vi "accelerometerChecker.vi"() -> ()   [LabVIEW 2021]
uses:
  <vilib>/DAQmx/read.llb/DAQmx Read (Analog 1D Wfm NChan NSamp).vi
  <vilib>/DAQmx/create/channels.llb/DAQmx Create Channel (AI-Voltage-Basic).vi
  <vilib>/DAQmx/create/channels.llb/DAQmx Create Channel (AI-Acceleration-Accelerometer).vi
  <vilib>/DAQmx/configure/timing.llb/DAQmx Timing (Sample Clock).vi
  <vilib>/DAQmx/miscellaneous.llb/DAQmx Fill In Error Info.vi
  <resource>/objmgr/daqmx.rc
panel:
  out "data 4":dynamicdata(graph) caption="data"
  out "data 3":dynamicdata(graph) caption="data"
  out "data 2":dynamicdata(graph) caption="data"
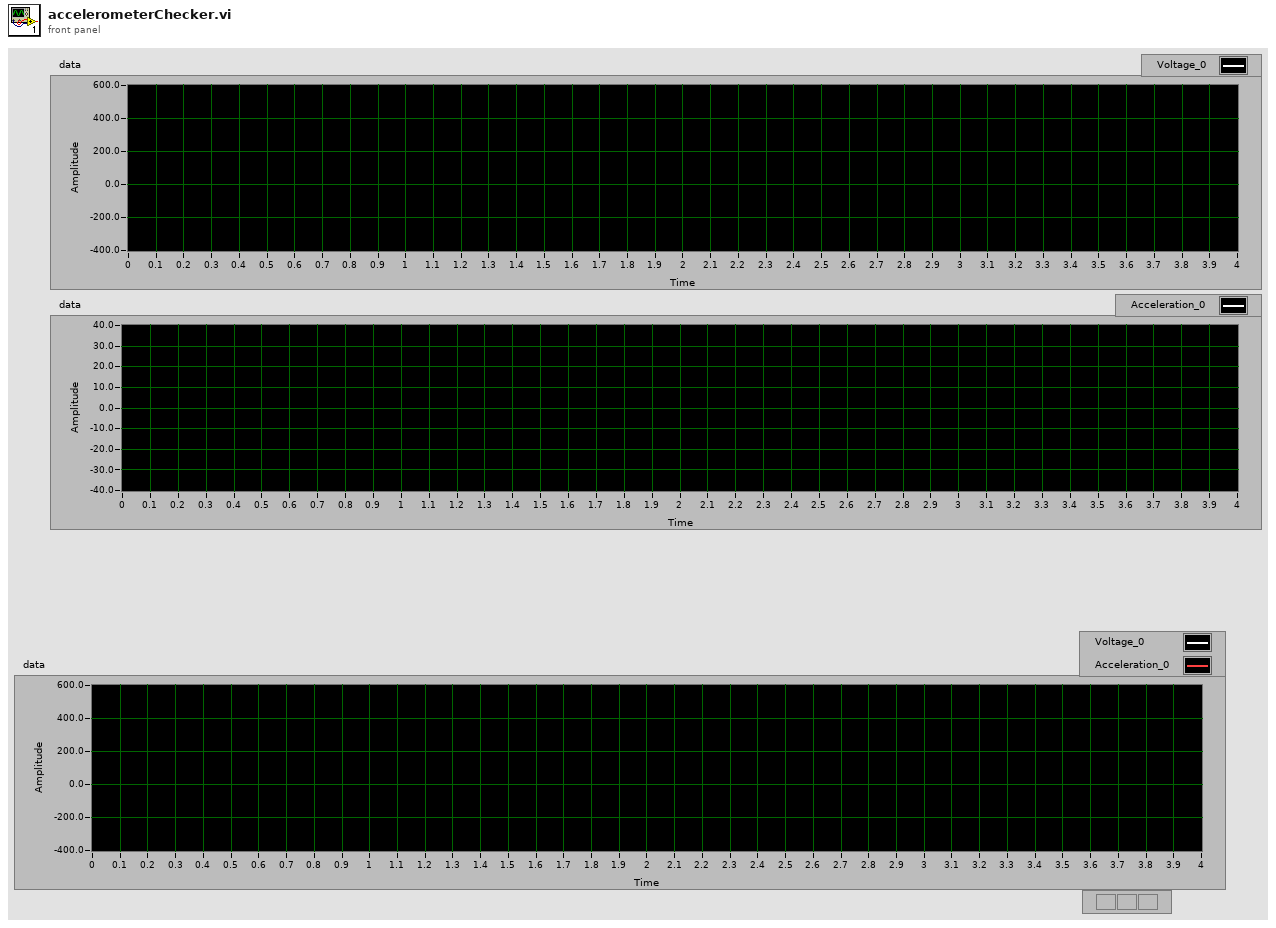
[diagram p1: front panel]
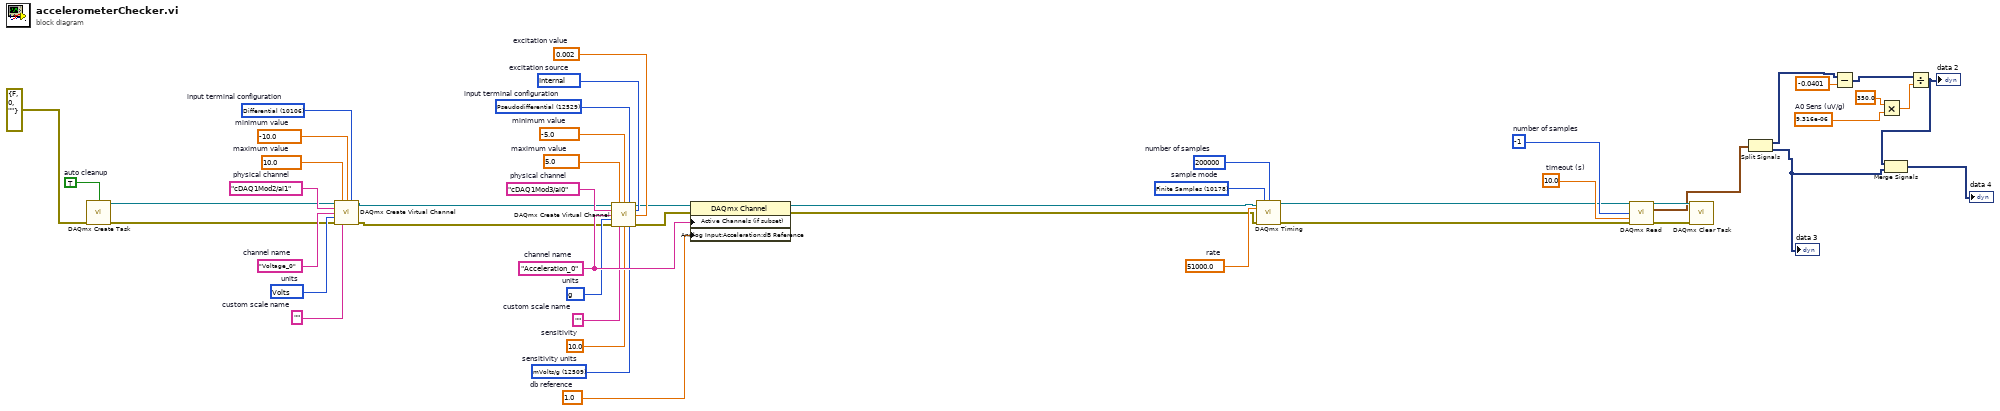
[diagram p0: block diagram]
diagram:
  w3 = 9.316e-06  # A0 Sens (uV/g)
  w29 = 1.0  # db reference
  w27 = 10186 items=["g"=10186, "m/s^2"=12470, "From Custom Scale"=10065]  # units
  w26 = 12529 items=["default"=-1, "RSE"=10083, "NRSE"=10078, "Differential"=10106, "Pseudodifferential"=12529]  # input terminal configuration
  w25 = 10200 items=["Internal"=10200, "External"=10167, "None"=10230]  # excitation source
  w24 = 0.002  # excitation value
  w23 = 12509 items=["mVolts/g"=12509, "Volts/g"=12510]  # sensitivity units
  w22 = 10.0  # sensitivity
  w30 = "Acceleration_0"  # channel name
  w20 = ""  # custom scale name
  w19 = -5.0  # minimum value
  w18 = 5.0  # maximum value
  w17 = "cDAQ1Mod3/ai0"  # physical channel
  w43 = 10178 items=["Finite Samples"=10178, "Continuous Samples"=10123, "Hardware Timed Single Point"=12522]  # sample mode
  w42 = 200000  # number of samples
  w41 = 51000.0  # rate
  w40 = 10106 items=["default"=-1, "RSE"=10083, "NRSE"=10078, "Differential"=10106, "Pseudodifferential"=12529]  # input terminal configuration
  w39 = 10348 items=["Volts"=10348, "From Custom Scale"=10065]  # units
  w38 = "Voltage_0"  # channel name
  w37 = ""  # custom scale name
  w36 = -10.0  # minimum value
  w35 = 10.0  # maximum value
  w34 = "cDAQ1Mod2/ai1"  # physical channel
  w32 = TRUE  # auto cleanup
  w47 = 10.0  # timeout (s)
  w48 = -1  # number of samples
  n1 = call <vilib>:"DAQmx Create Task.vi"("auto cleanup"=w32, "error in"=errorcluster {"status"=FALSE, "code"=0, "source"=""}) -> ("task out"=w33:refnum<k21>, "error out"=w31:errorcluster)  [unwired: 12 in]
  n2 = call-poly <vilib>:"DAQmx Create Virtual Channel.vi"("task in"=w33, "maximum value"=w35, "minimum value"=w36, "input terminal configuration"=w40, "physical channels"=w34, "name to assign"=w38, "units"=w39, "error in"=w31, "custom scale name"=w37) -> ("task out"=w16:refnum<k21>, "error out"=w15:errorcluster)  [unwired: 5 in]
  n3 = call-poly <vilib>:"DAQmx Create Virtual Channel.vi"("task in"=w16, "maximum value"=w18, "minimum value"=w19, "input terminal configuration"=w26, "physical channels"=w17, "current excitation source"=w25, "name to assign"=w30, "current excitation value"=w24, "units"=w27, "error in"=w15, "custom scale name"=w20, "sensitivity"=w22, "sensitivity units"=w23) -> ("task out"=w21:refnum<k21>, "error out"=w28:errorcluster)  [unwired: 1 in]
  n4 = property class="DAQmx Channel"(reference=w21, error in=w28, "Active Channels (if subset)"=w30, "Analog Input:Acceleration:dB Reference"=w29) -> (reference out=w14:refnum<k21>, error out=w13:errorcluster)
  n5 = call-poly <vilib>:"DAQmx Timing.vi"("task/channels in"=w14, "sample mode"=w43, "samples per channel"=w42, "rate"=w41, "error in"=w13) -> ("task out"=w12:refnum<k21>, "error out"=w11:errorcluster)  [unwired: 9 in]
  n6 = call-poly <vilib>:"DAQmx Read.vi"("task/channels in"=w12, "number of samples per channel"=w48, "timeout"=w47, "error in"=w11) -> ("task out"=w45:refnum<k21>, "data"=w10:waveform(dbl)[], "error out"=w46:errorcluster)  [unwired: 9 in]
  n7 = call <vilib>:"DAQmx Clear Task.vi"("task in"=w45, "error in"=w46) -> ()  [unwired: 13 in, 1 out]
  n8 = Split Signals(w10) -> (w5:dynamicdata, w8:dynamicdata)  [unwired: 2 in]
  "data 3" <- w8
  n9 = Subtract(x=w5, y=-0.0401) -> (x-y=w1:dynamicdata)
  n10 = Multiply(x=350.0, y=w3) -> (x*y=w2:dbl)
  n11 = Divide(x=w1, y=w2) -> (x/y=w4:dynamicdata)
  "data 2" <- w4
  n12 = Merge Signals(w4, w8) -> (→"data 4":dynamicdata)
